vi "LinearMove.vi"(0 "Time":fxp<+,64,64>, 1 "Start":i16, 4 "End":i16, 5 "Velocity":fxp<+/-,16,16>, 8 "ExpandVelScaller":i16=-27) -> (14 "OutPosition":i16, 19 "Finished Move":bool)   [LabVIEW 2023]
uses:
  <vilib>/rvi/Arithmetic/AddSubMult/XNode/nirviSatArithmetic.xnode
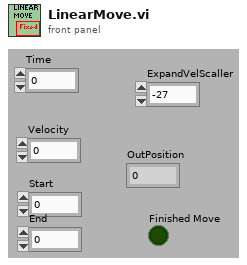
[diagram p1: front panel]
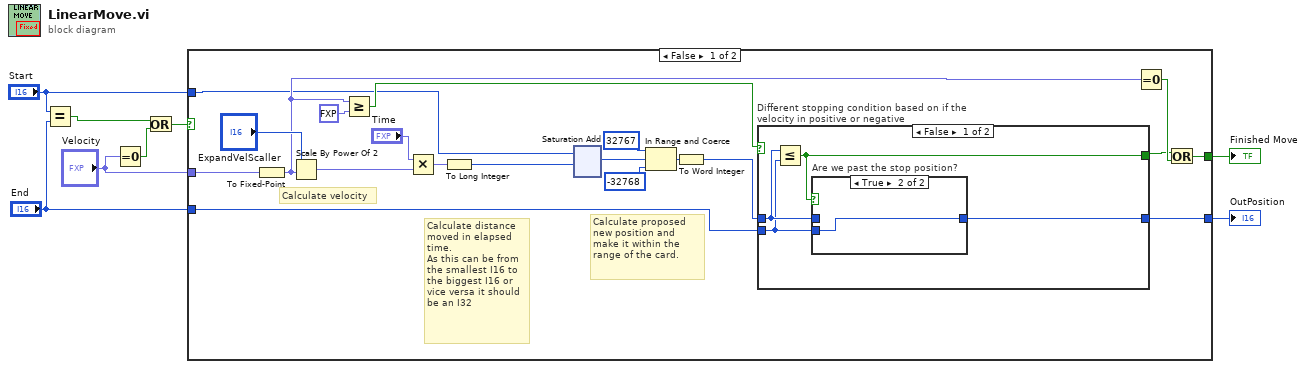
[diagram p0: block diagram]
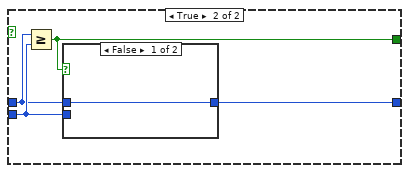
[diagram p3: hidden frame]
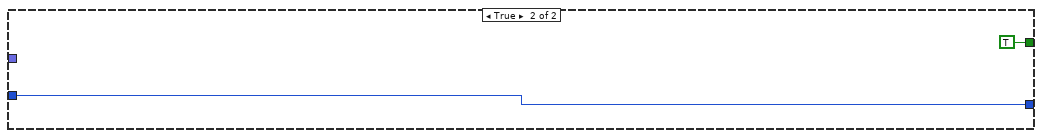
[diagram p5: hidden frame]
diagram:
  n1 = Equal?(x="Start", y="End") -> (x = y?=w4:bool)
  n2 = Equal To 0?(x="Velocity") -> (x = 0?=w3:bool)
  n3 = Or(x=w4, y=w3) -> (x .or. y?=w2:bool)
  n4 = case shown="False" w2 {
    tunnel: [w27 TRUE] -> w8
    tunnel: "Velocity" -> [w18 _]
    tunnel: [w17 w60] -> w1
    tunnel: "End" -> [w16 w60]
    tunnel: "Start" -> [w14 _]
    frame False {
      # "Calculate proposed new position and make it within the range of the card."
      # "Calculate distance moved in elapsed time.\nAs this can be from the smallest I16 to the biggest I16 or vice versa it should be an I32"
      # "Calculate velocity"
      n5 = To Fixed-Point(number=w18) -> (fixed-point=w20:fxp<+/-,48,16>)  [unwired: 1 in]
      n6 = Scale By Power Of 2(n="ExpandVelScaller", x=w20) -> (x*2^n=w22:fxp<+/-,48,16>)
      n7 = Greater Or Equal?(x=w20, y=fxp<+,1,1> 0.0) -> (x >= y?=w25:bool)
      n8 = Multiply(x="Time", y=w22) -> (x*y=w21:fxp<+/-,64,64>)
      n9 = To Long Integer(number=w21) -> (32bit integer=w13:i32)
      n10 = xnode "Saturation Add"("x"=w14, "y"=w13) -> ("x+y"=w12:i32)  [unwired: 1 out]
      n11 = In Range and Coerce(upper limit=32767, x=w12, lower limit=-32768) -> (coerced(x)=w11:i32)  [unwired: 1 out]
      n12 = To Word Integer(number=w11) -> (16bit integer=w15:i16)
      n13 = case "Different stopping condition based on if the velocity in positive or negative" shown="False" w25 {
        tunnel: w15 -> [w49 w54]
        tunnel: w16 -> [w48 w55]
        tunnel: [w50 w56] -> w17
        tunnel: [w47 w53] -> w19
        frame False {
          n14 = Less Or Equal?(x=w49, y=w48) -> (x <= y?=w47:bool)
          n15 = case "Are we past the stop position?" shown="True" w47 {
            tunnel: [w51 w52] -> w50
            tunnel: w48 -> [_ w52]
            tunnel: w49 -> [w51 _]
            frame False {
            }
            frame True {
            }
          }
        }
        frame True {
          n16 = Greater Or Equal?(x=w54, y=w55) -> (x >= y?=w53:bool)
          n17 = case shown="False" w53 {
            tunnel: w55 -> [_ w58]
            tunnel: [w57 w58] -> w56
            tunnel: w54 -> [w57 _]
            frame False {
            }
            frame True {
            }
          }
        }
      }
      n18 = Equal To 0?(x=w20) -> (x = 0?=w28:bool)
      n19 = Or(x=w19, y=w28) -> (x .or. y?=w27:bool)
    }
    frame True {
    }
  }
  "Finished Move" <- w8
  "OutPosition" <- w1
